vi "纬度.vi"(11 "纬度":string) -> (1 "纬度方向":string, 2 "纬分":dbl, 3 "纬度":i32)   [LabVIEW 2018]
panel:
  out "数字":i32
  out "数值":i32
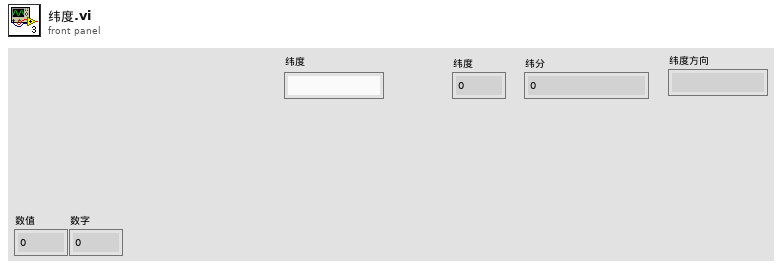
[diagram p1: front panel]
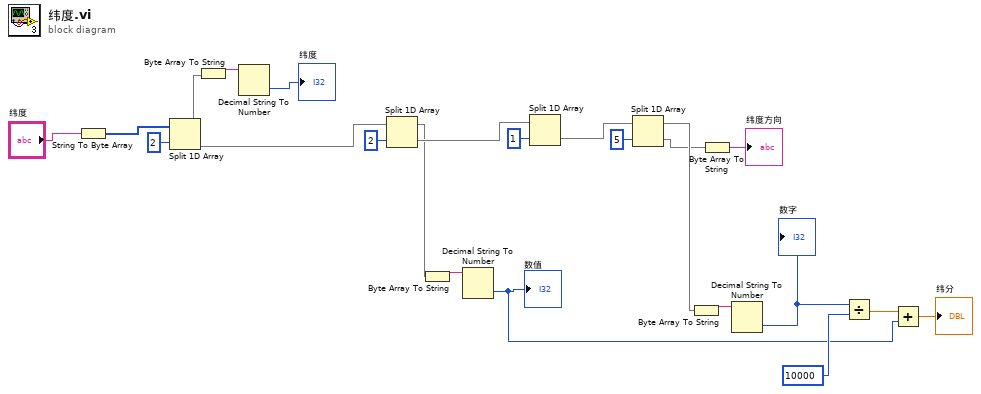
[diagram p0: block diagram]
diagram:
  n1 = String To Byte Array(string="纬度") -> (unsigned byte array=w22:u8[])
  n2 = Split 1D Array(array=w22, index=2 ("索引")) -> (first subarray=w20:u8[], second subarray=w19:u8[])
  n3 = Byte Array To String(unsigned byte array=w20) -> (string=w14:string)
  n4 = Decimal String To Number(string=w14) -> (number=→"纬度":i32)  [unwired: 2 in, 1 out]
  n5 = Split 1D Array(array=w19, index=2 ("索引")) -> (first subarray=w9:u8[], second subarray=w17:u8[])
  n6 = Byte Array To String(unsigned byte array=w9) -> (string=w11:string)
  n7 = Decimal String To Number(string=w11) -> (number=w2:i32)  [unwired: 2 in, 1 out]
  "数值" <- w2
  n8 = Split 1D Array(array=w17, index=1 ("索引")) -> (second subarray=w15:u8[])  [unwired: 1 out]
  n9 = Split 1D Array(array=w15, index=5 ("索引")) -> (first subarray=w8:u8[], second subarray=w7:u8[])
  n10 = Byte Array To String(unsigned byte array=w8) -> (string=w10:string)
  n11 = Byte Array To String(unsigned byte array=w7) -> (string=→"纬度方向":string)
  n12 = Decimal String To Number(string=w10) -> (number=w5:i32)  [unwired: 2 in, 1 out]
  "数字" <- w5
  n13 = Divide(x=w5, y=10000) -> (x/y=w3:dbl)
  n14 = Add(x=w3, y=w2) -> (x+y=→"纬分":dbl)
